vi "Calculate Integral.vi"(9 "Right Boundary Array":dbl[](array[numeric]), 10 "Left Boundary Array":dbl[](array[numeric]), 11 "Waveform":waveform(dbl)) -> (2 "Maximums":dbl[](array[numeric]), 3 "Integrals":dbl[](array[numeric]))   [LabVIEW 2014, in "MassSpectrumExtractor.lvclass"]
uses:
  MassSpectrumExtractor.lvclass
  <vilib>/Waveform/WDTOps.llb/WDT Get Waveform Subset DBL.vi
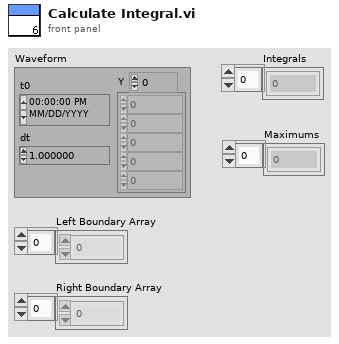
[diagram p1: front panel]
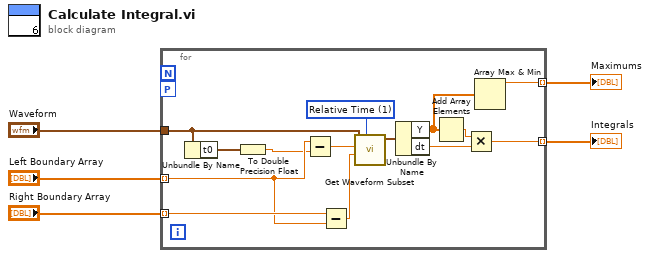
[diagram p0: block diagram]
diagram:
  n1 = for {
    tunnel: "Right Boundary Array" -> [w18] mode=indexing
    tunnel: "Left Boundary Array" -> [w10] mode=indexing
    tunnel: "Waveform" -> [w12]
    tunnel: [w14] -> w5 mode=indexing
    workers-P: _ -> [_]
    tunnel: [w6] -> w1 mode=indexing
    w13 = u16 1 items=["Samples", "Relative Time"] ("start/duration format")
    n2 = Unbundle By Name(w12) -> ("t0"=w11:timestamp)
    n3 = To Double Precision Float(number=w11) -> (double precision float=w9:dbl)
    n4 = Subtract(x=w10, y=w9) -> (x-y=w8:dbl)
    n5 = Subtract(x=w18, y=w10) -> (x-y=w19:dbl)
    n6 = call-poly <vilib>:"Get Waveform Subset.vi"("start/duration format"=w13, "duration"=w19, "start samples/time"=w8, "waveform in"=w12) -> ("waveform out"=w17:waveform(dbl))  [unwired: 2 in, 3 out]
    n7 = Unbundle By Name(w17) -> ("Y"=w7:dbl[], "dt"=w15:dbl)
    n8 = Add Array Elements(numeric array=w7) -> (sum=w16:dbl)
    n9 = Multiply(x=w16, y=w15) -> (x*y=w14:dbl)
    n10 = Array Max & Min(array=w7) -> (max value=w6:dbl)  [unwired: 3 out]
  }
  "Integrals" <- w5
  "Maximums" <- w1
